vi "Message Queue VIs.vi"   [LabVIEW 2014]
uses:
  vilib/Message/Msg Post UI Message.vi
  vilib/Message/Msg Send UI Message.vi
  vilib/Message/Msg Post Priority UI Message.vi
  vilib/Message/Msg Send Priority UI Message.vi
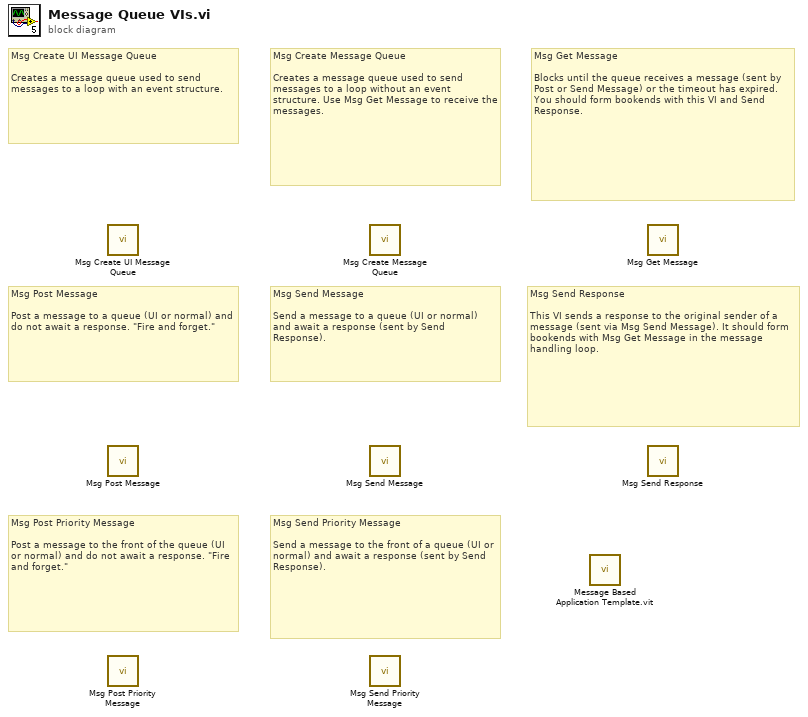
[diagram p0: block diagram]
diagram:
  # "Msg Send Response\n\nThis VI sends a response to the original sender of a message (sent via Msg Send Message). It should form bookends with Msg Get Message in the message handling loop."
  # "Msg Send Priority Message\n\nSend a message to the front of a queue (UI or normal) and await a response (sent by Send Response)."
  # "Msg Post Priority Message\n\nPost a message to the front of the queue (UI or normal) and do not await a response. \"Fire and forget.\""
  # "Msg Send Message\n\nSend a message to a queue (UI or normal) and await a response (sent by Send Response)."
  # "Msg Post Message\n\nPost a message to a queue (UI or normal) and do not await a response. \"Fire and forget.\""
  # "Msg Get Message\n\nBlocks until the queue receives a message (sent by Post or Send Message) or the timeout has expired. You should form bookends with this VI and Send Response."
  # "Msg Create Message Queue\n\nCreates a message queue used to send messages to a loop without an event structure. Use Msg Get Message to receive the messages."
  # "Msg Create UI Message Queue\n\nCreates a message queue used to send messages to a loop with an event structure."
  n1 = call "Msg Create UI Message Queue.vi"() -> ()  [unwired: 7 in, 3 out]
  n2 = call-poly "Msg Post Message.vi"() -> ()  [unwired: 7 in, 3 out]
  n3 = call-poly "Msg Post Priority Message.vi"() -> ()  [unwired: 8 in, 2 out]
  n4 = call "Msg Create Message Queue.vi"() -> ()  [unwired: 7 in, 3 out]
  n5 = call-poly "Msg Send Message.vi"() -> ()  [unwired: 6 in, 4 out]
  n6 = call-poly "Msg Send Priority Message.vi"() -> ()  [unwired: 8 in, 2 out]
  n7 = call "Message Based Application Template.vit"() -> ()  [unwired: 1 in]
  n8 = call "Msg Get Message.vi"() -> ()  [unwired: 4 in, 5 out]
  n9 = call "Msg Send Response.vi"() -> ()  [unwired: 9 in, 1 out]
